vi "DAQ_DC-RMS Current Meas Initialize.vi"(0 "Physical Channels":tag, 7 "Global Channels":refnum<k21>, 11 "error in":errorcluster) -> (4 "DAQmx Task Out":refnum<k21>, 15 "error out":errorcluster)   [LabVIEW 2021, in "DAQ_DC-RMS Current Measurement.lvlib"]
doc: "Initialize analog input channels and obtains a DAQmx task\n\nProvide either Physical channel or Global Channel\nIf both physical and Global channels are provided, Global Channels will take precedence\n\nNote: Global channel(s) should be declared as AI Current."
uses:
  DAQ_DC-RMS Current Measurement.lvlib
  <vilib>/DAQmx/create/channels.llb/DAQmx Create Channel (AI-Current-Basic).vi
panel:
  # "Inputs"
  # "Outputs"
  # "Overview:\nThis VI initializes an analog input and provides the DAQmx Task Out\n\nHardware Requirement: A compatible PXI, PCIe, USB, cDAQ or Testscale device\n\nSoftware Requirement: NI DAQmx 2022 Q4 or later\n\nInstructions:\n1. Enter physical channel in which DC Current Measurement has to be done in Physical Channels control. (Or) Enter Global channels to use it instead of initiating a new task. Note: Global channel(s) should be declared as AI Current.\n2. User must configure only one input. If both are mentioned, Global Channels will take precedence.\n3. Get the DC Current Measurement task from DAQmx Task Out\n\nNote: User can use the DAQmx Task on other VIs to configure and initiate DC Current and Measurements."
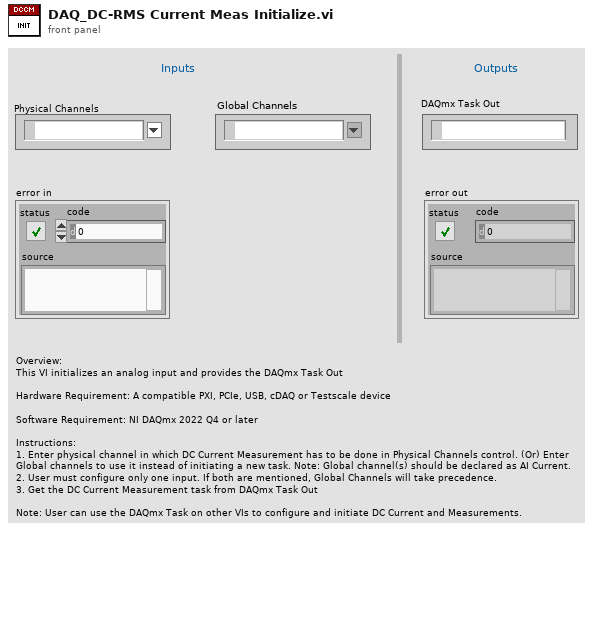
[diagram p1: front panel]
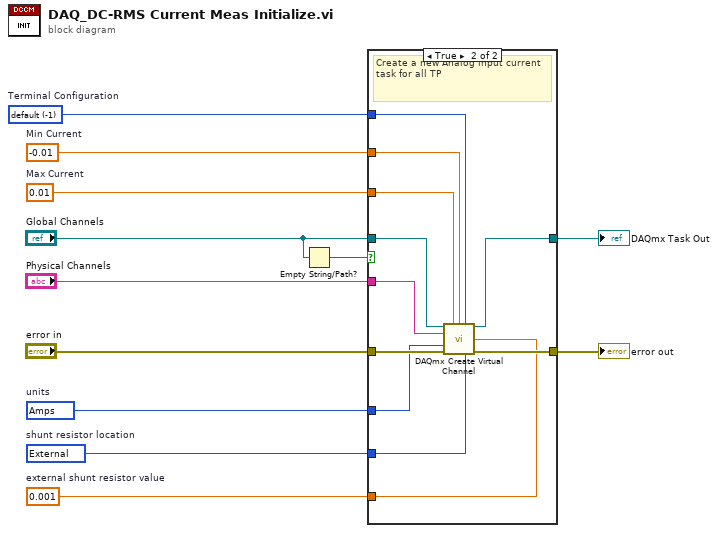
[diagram p0: block diagram]
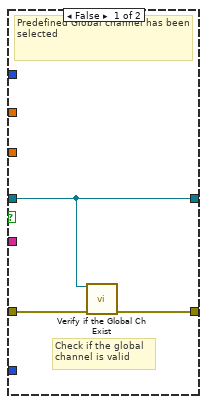
[diagram p2: hidden frame]
diagram:
  w3 = 0.001  # external shunt resistor value
  w4 = 10167 items=["default"=-1, "Internal"=10200, "External"=10167]  # shunt resistor location
  w5 = 10342 items=["Amps"=10342, "From Custom Scale"=10065]  # units
  w6 = -1 items=["default"=-1, "RSE"=10083, "NRSE"=10078, "Differential"=10106, "Pseudodifferential"=12529]  # Terminal Configuration
  w7 = -0.01  # Min Current
  w8 = 0.01  # Max Current
  n1 = Empty String/Path?(string/path="Global Channels") -> (empty?=w2:bool)
  n2 = case shown="True" w2 {
    tunnel: "Physical Channels" -> [_ w23]
    tunnel: "Global Channels" -> [w13 w26]
    tunnel: [w13 w25] -> w9
    tunnel: "error in" -> [w15 w24]
    tunnel: [w14 w22] -> w12
    tunnel: w8 -> [_ w21]
    tunnel: w7 -> [_ w20]
    tunnel: w6 -> [_ w19]
    tunnel: w5 -> [_ w18]
    tunnel: w4 -> [_ w17]
    tunnel: w3 -> [_ w16]
    frame False {
      # "Check if the global\nchannel is valid"
      # "Predefined Global channel has been selected"
      n3 = call "Verify if the Global Ch Exist.vi"("Global Channels"=w13, "error in (no error)"=w15) -> ("error out"=w14:errorcluster)  [unwired: 13 in]
    }
    frame True {
      # "Create a new Analog input current task for all TP"
      n4 = call-poly <vilib>:"DAQmx Create Virtual Channel.vi"("task in"=w26, "maximum value"=w21, "minimum value"=w20, "input terminal configuration"=w19, "physical channels"=w23, "external shunt resistor value"=w16, "units"=w18, "error in"=w24, "shunt resistor location"=w17) -> ("task out"=w25:refnum<k21>, "error out"=w22:errorcluster)  [unwired: 5 in]
    }
  }
  "DAQmx Task Out" <- w9
  "error out" <- w12
